vi "TrajectoryState_GetAll.vi"(11 "TRAJ_STATE":T1={"TimeSeconds"=0.0, "Velocity"=0.0, "Acceleration"=0.0, "POSE"={"TRANSLATION"={"X"=0.0, "Y"=0.0}, "ROTATION"={"VALUE"=0.0, "COS"=1.0, "SIN"=0.0}}, "Curvature"=0.0} {"POSE"."ROTATION"."SIN" format="%13.4f"; "POSE"."ROTATION"."COS" format="%13.4f"; "POSE"."ROTATION"."VALUE" format="%13.4f"; "POSE"."TRANSLATION"."Y" format="%14.3f"; "POSE"."TRANSLATION"."X" format="%14.3f"}) -> (0 "Heading":dbl, 1 "Y":dbl, 2 "X":dbl, 3 "Curvature":dbl, 4 "TimeSeconds":dbl, 5 "Acceleration":dbl, 7 "Velocity":dbl)   [LabVIEW 2019, in "Trajectory_Library.lvlib"]
doc: "Get individual items from the trajectory state cluster\n \nParameters:\n - TrajState - TrajectoryState data structure\n \nReturns:\n - Velocity -- chassis velocity M/S\n - Acceleration -- chassis accleration M/S^2\n - Curvature -- chassis curvature RADIAN/METER\n - X -- chassis X position M\n - Y -- chassis Y position M\n - Heading -- chassis heading RADIANS\n - Time -- Sample time SECONDS"
uses:
  TRAJ_STATE.ctl
  POSE2D.ctl
  TRANSLATION2D.ctl
  ROTATION2D.ctl
  Trajectory_Library.lvlib
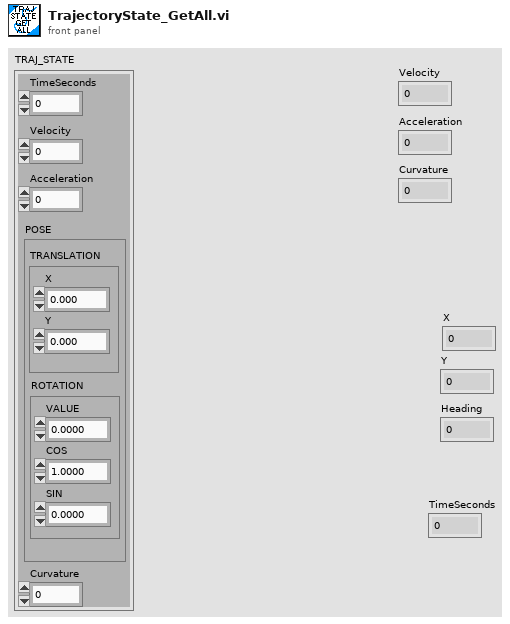
[diagram p1: front panel]
types:
  T1 = typedef "Trajectory_Library.lvlib/TRAJ_STATE.ctl" = cluster{"TimeSeconds":dbl, "Velocity":dbl, "Acceleration":dbl, "POSE":T2, "Curvature":dbl}
  T2 = typedef "Trajectory_Library.lvlib/POSE2D.ctl" = cluster{"TRANSLATION":T3, "ROTATION":T4}
  T3 = typedef "Trajectory_Library.lvlib/TRANSLATION2D.ctl" = cluster{"X":dbl, "Y":dbl}
  T4 = typedef "Trajectory_Library.lvlib/ROTATION2D.ctl" = cluster{"VALUE":dbl, "COS":dbl, "SIN":dbl}
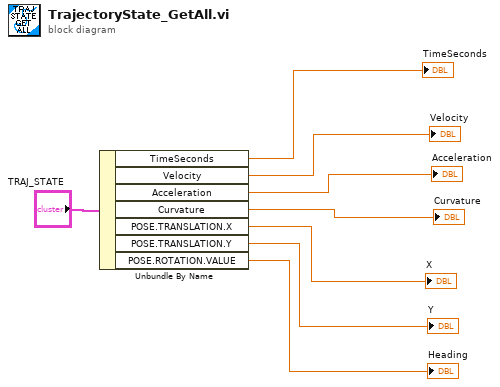
[diagram p0: block diagram]
diagram:
  n1 = Unbundle By Name("TRAJ_STATE") -> ("TimeSeconds"=→"TimeSeconds":dbl, "Velocity"=→"Velocity":dbl, "Acceleration"=→"Acceleration":dbl, "Curvature"=→"Curvature":dbl, "POSE.TRANSLATION.X"=→"X":dbl, "POSE.TRANSLATION.Y"=→"Y":dbl, "POSE.ROTATION.VALUE"=→"Heading":dbl)
